vi "XboxTeleop.vi"(10 "Match Info":T1={"Autonomous Elapsed Seconds"=0.0, "TeleOp Elapsed Seconds"=0.0, "Disabled Elapsed Seconds"=0.0, "Visited Autonomous"=FALSE, "Visited TeleOp"=FALSE, "Visited Disabled"=FALSE, "Autonomous Settings"={"Autonomous Style"=enum."Independent", "VI Refnum"=refnum}}, 11 "Call Context":T2) -> ()   [LabVIEW 2015]
doc: "This VI is called for each TeleOp packet received from the DS where the robot is not disabled. It is often used to read from the joysticks and update I/O or to update setpoints for timed control loops. It should complete and return within 20 milliseconds or it may miss DS packets."
uses:
  <vilib>/Rock Robotics/WPI/DriverStation/WPI_DriverStationDerivedRobotMode.ctl
  <vilib>/Rock Robotics/WPI/DriverStation/WPI_DriverStationMatch Info.ctl
  <vilib>/Rock Robotics/WPI/Utilities/WPI_GetSetVariantRefNum.vi
  <vilib>/Rock Robotics/Network Tables/NT Write Boolean Array.vi
  <vilib>/Rock Robotics/Network Tables/NT Write Numeric Array.vi
  <vilib>/Rock Robotics/Network Tables/NT Write Boolean.vi
  <vilib>/Rock Robotics/Network Tables/NT Read Boolean.vi
  <vilib>/Rock Robotics/Network Tables/NT Read Number.vi
  <vilib>/Rock Robotics/WPI/RobotDrive/WPI_RobotDriveArcadeDrive_Standard(NoSaturation).vi
panel:
  in  "TurnPercent":dbl=0.9 format="%#_13g"
  out "TurnOutput":dbl(slide) scale=-1.0..1.0
  out "MotorInput":dbl(knob) scale=-1.0..1.0
  in  "DrivePercent":dbl=0.75 format="%#_13g"
  out "Sample Slider 0":dbl(slide) scale=0.0..5.0
  out "Sample Boolean 1":bool
  out "Sample Boolean 0":bool
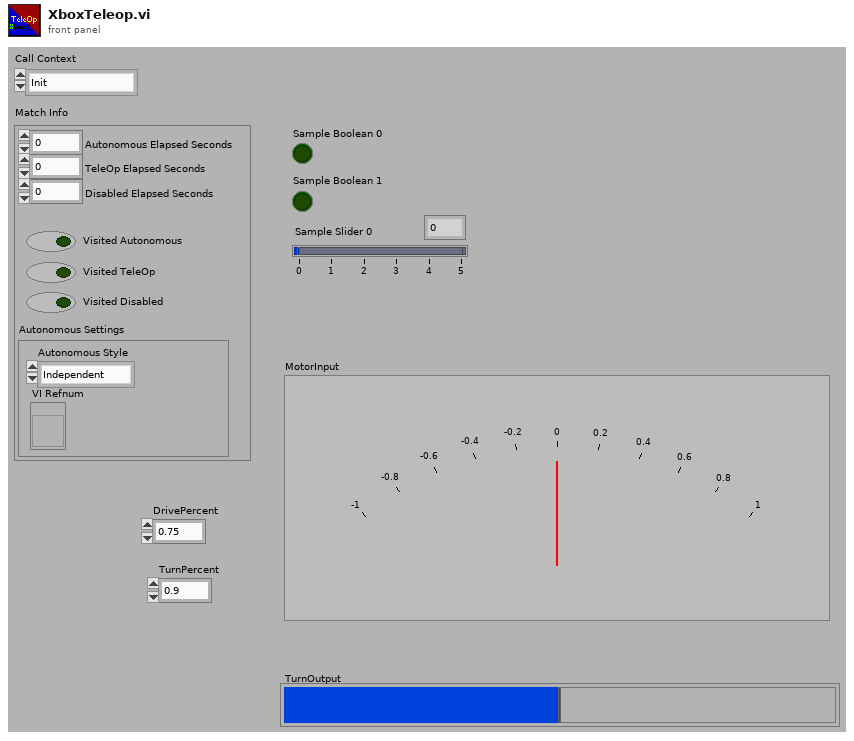
[diagram p1: front panel]
types:
  T1 = typedef "WPI_DriverStationMatch Info.ctl" = cluster{"Autonomous Elapsed Seconds":dbl, "TeleOp Elapsed Seconds":dbl, "Disabled Elapsed Seconds":dbl, "Visited Autonomous":bool, "Visited TeleOp":bool, "Visited Disabled":bool, "Autonomous Settings":cluster{"Autonomous Style":enum16{"Iterative", "Independent"}, "VI Refnum":refnum<vi>}}
  T2 = typedef "WPI_DriverStationDerivedRobotMode.ctl" = enum16{"Init", "Execute", "Stop"}
  T3 = typedef "WPI_RobotDriveDevRef.ctl" = cluster{"DevStatus":errorcluster, "Motors[]":T4[], "Square Inputs":bool, "Max Output":dbl}
  T4 = typedef "WPI_MotorControlDeviceRef.ctl" = cluster{"DeviceStatus":errorcluster, "Type":T5, "PWM":cluster{"PWM Channel":T6, "DeadBand":T7}, "CAN":cluster{"Device Number":u8, "Control Mode":T8, "Semaphore":T9, "Max Vout":dbl, "TalonSRX Control Mode":T10}, "Invert":bool}
  T5 = typedef "WPI_MotorControlType.ctl" = enum16{"PWM", "CAN", "CANTalonSRX"}
  T6 = typedef "FPGA_DIOPWMChannel.ctl" = enum8{"PWM 0", "PWM 1", "PWM 2", "PWM 3", "PWM 4", "PWM 5", "PWM 6", "PWM 7", "PWM 8", "PWM 9", "PWM MXP 0", "PWM MXP 1", "PWM MXP 2", "PWM MXP 3", "PWM MXP 4", "PWM MXP 5", "PWM MXP 6", "PWM MXP 7", "PWM MXP 8", "PWM MXP 9", "Invalid"}
  T7 = typedef "WPI_PWMDeadband.ctl" = cluster{"Name":string, "maxPositivePwm":i32, "minPositivePwm":i32, "centerPwm":i32, "maxNegativePwm":i32, "minNegativePwm":i32, "angularRange":u16}
  T8 = typedef "WPI_CANJaguar_ControlMode.ctl" = enum8{"Percent VBus", "Current", "Speed", "Position", "Voltage"}
  T9 = typedef "Semaphore RefNum" = refnum<k1>
  T10 = typedef "WPI_CANTalonSRX_APIControlMode.ctl" = enum8{"Percent VBus", "Speed", "Position", "Slave", "Unchanged / Invalid", "Voltage Compensation", "Current", "Motion Profile"}
  T11 = typedef "WPI_JoystickDevRef.ctl" = cluster{"Device":T12}
  T12 = typedef "WPI_JoystickDeviceEnum.ctl" = enum16{"USB 0", "USB 1", "USB 2", "USB 3", "USB 4", "USB 5"}
  T13 = cluster{"Buttons[0]":bool, "Buttons[1]":bool, "Buttons[2]":bool, "Buttons[3]":bool, "Buttons[4]":bool, "Buttons[5]":bool, "Buttons[6]":bool, "Buttons[7]":bool, "Buttons[8]":bool}
  T14 = cluster{"Axes[0]":dbl, "Axes[1]":dbl, "Axes[2]":dbl, "Axes[3]":dbl, "Axes[4]":dbl, "Axes[5]":dbl, "Axes[6]":dbl, "Axes[7]":dbl, "Axes[8]":dbl}
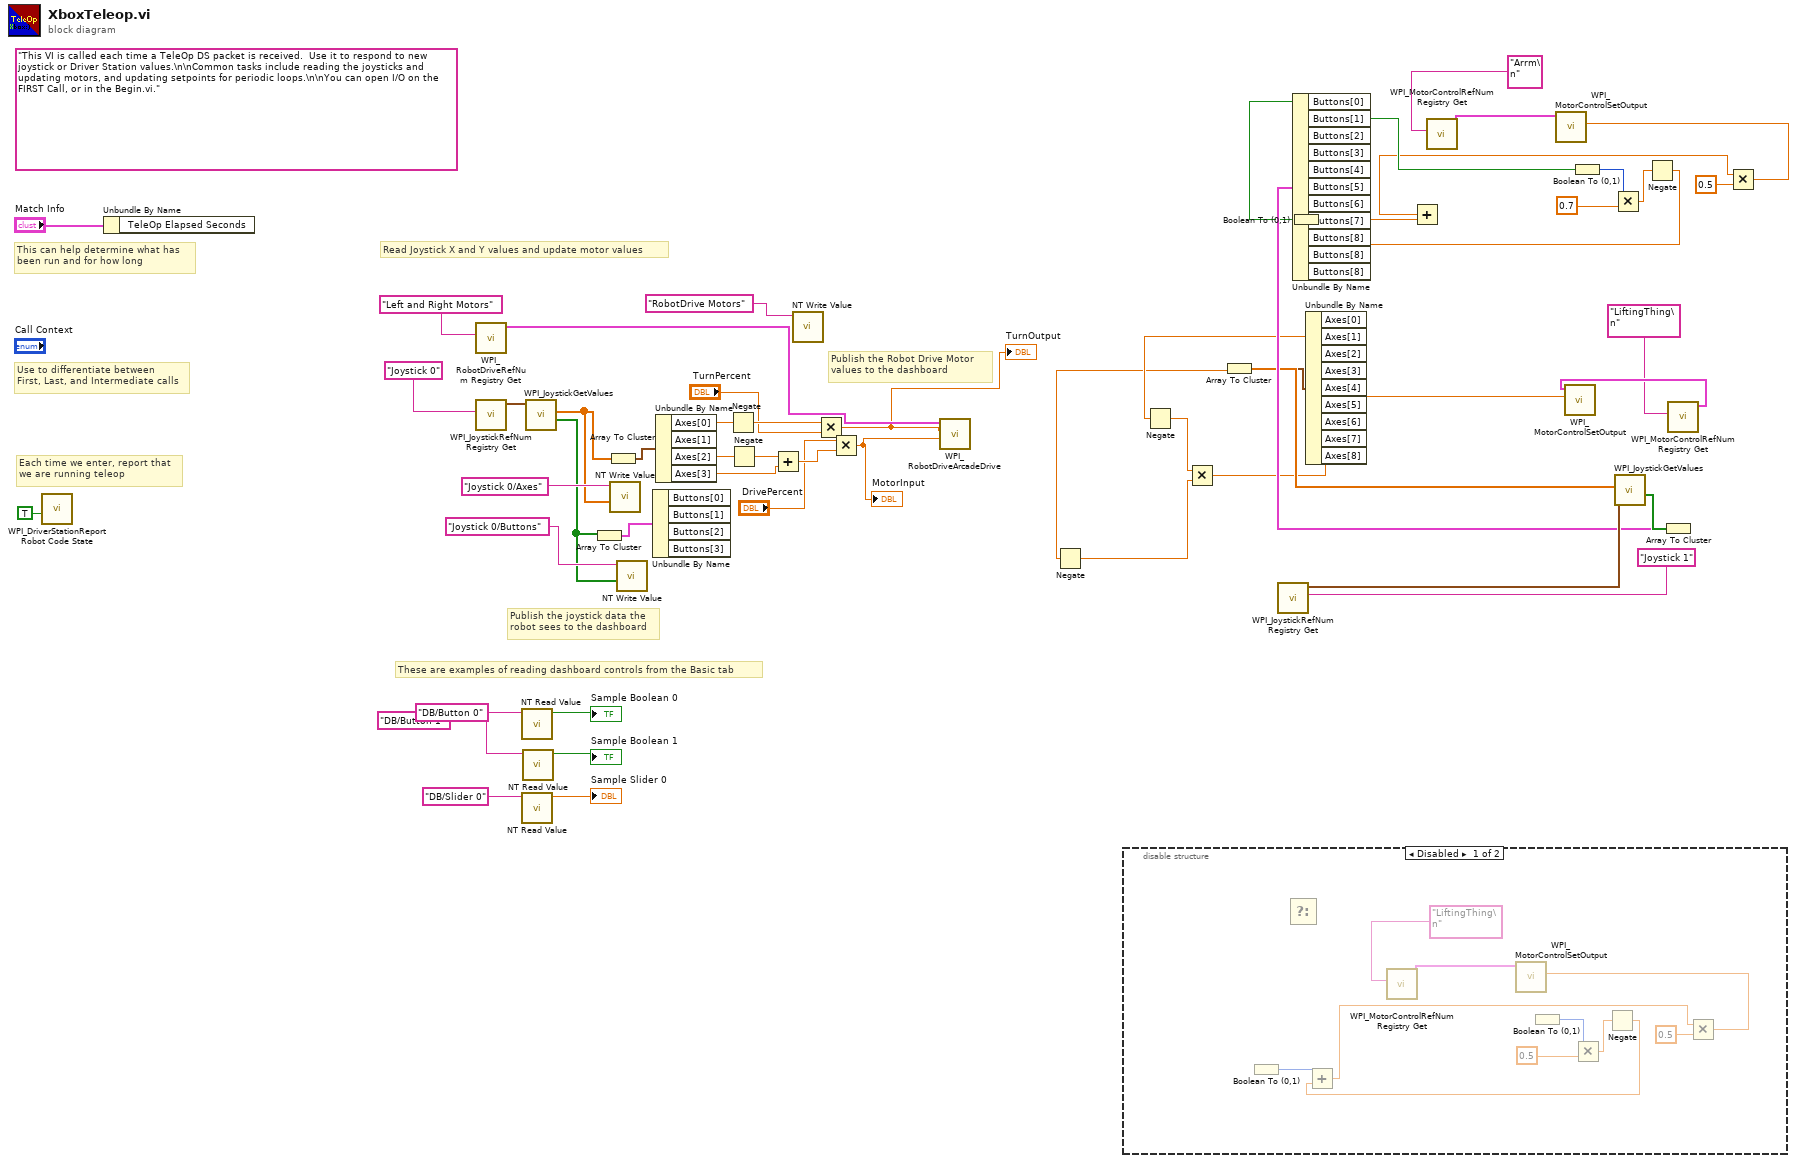
[diagram p0: block diagram]
diagram:
  (unwired) "This VI is called each time a TeleOp DS packet is received.  Use it to respond to new joystick or Driver Station values.\n\nCommon tasks include reading the joysticks and updating motors, and updating setpoints for periodic loops.\n\nYou can open I/O on the FIRST Call, or in the Begin.vi."
  # "These are examples of reading dashboard controls from the Basic tab"
  # "Publish the Robot Drive Motor\nvalues to the dashboard"
  # "Publish the joystick data the\nrobot sees to the dashboard"
  # "Each time we enter, report that\nwe are running teleop"
  # "Use to differentiate between\nFirst, Last, and Intermediate calls"
  # "This can help determine what has\nbeen run and for how long"
  # "Read Joystick X and Y values and update motor values"
  n1 = call <vilib>:"WPI_DriverStationReport Robot Code State.vi"("TeleOp"=TRUE ("Autonomous")) -> ()  [unwired: 10 in, 1 out]
  n2 = Unbundle By Name("Match Info") -> ()  [unwired: 1 out]
  n3 = call <vilib>:"WPI_RobotDriveRefNum Registry Get.vi"("refnum name"="Left and Right Motors") -> ("RobotDriveDevRef"=w38:T3)  [unwired: 1 in, 9 out]
  n4 = call <vilib>:"WPI_JoystickRefNum Registry Get.vi"("refnum name"="Joystick 0") -> ("JoystickDevRef"=w51:T11)  [unwired: 1 in, 9 out]
  n5 = call-poly <vilib>:"NT Read Value.vi"("Name"="DB/Button 0" ("refnum name")) -> ("Boolean"=→"Sample Boolean 0":bool)  [unwired: 9 in, 1 out]
  n6 = call-poly <vilib>:"NT Read Value.vi"("Name"="DB/Slider 0" ("refnum name")) -> ("Numeric"=→"Sample Slider 0":dbl)  [unwired: 9 in, 1 out]
  n7 = call-poly <vilib>:"NT Read Value.vi"("Name"="DB/Button 1" ("refnum name")) -> ("Boolean"=→"Sample Boolean 1":bool)  [unwired: 9 in, 1 out]
  n8 = call <vilib>:"WPI_JoystickGetValues.vi"("JoystickDevRef"=w51) -> ("Buttons"=w36:bool[], "Axes"=w39:dbl[])  [unwired: 6 in, 3 out]
  n9 = Array To Cluster(array=w36) -> (cluster=w35:T13)
  n10 = Array To Cluster(array=w39) -> (cluster=w40:T14)
  n11 = call-poly <vilib>:"NT Write Value.vi"("Numeric Array"=w39, "Name"="Joystick 0/Axes") -> ()  [unwired: 9 in, 1 out]
  n12 = call-poly <vilib>:"NT Write Value.vi"("Boolean Array"=w36, "Name"="Joystick 0/Buttons") -> ()  [unwired: 9 in, 1 out]
  n13 = Unbundle By Name(w35) -> ()  [unwired: 4 out]
  n14 = Unbundle By Name(w40) -> ("Axes[0]"=w37:dbl, "Axes[2]"=w34:dbl, "Axes[3]"=w32:dbl)  [unwired: 1 out]
  n15 = Negate(x=w37) -> (-x=w29:dbl)
  n16 = Negate(x=w34) -> (-x=w33:dbl)
  n17 = Add(x=w33, y=w32) -> (x+y=w31:dbl)
  n18 = call-poly <vilib>:"NT Write Value.vi"("Name"="RobotDrive Motors") -> ()  [unwired: 10 in, 1 out]
  n19 = Multiply(x=w29, y="TurnPercent") -> (x*y=w28:dbl)
  "TurnOutput" <- w28
  n20 = Multiply(x="DrivePercent", y=w31) -> (x*y=w30:dbl)
  "MotorInput" <- w30
  n21 = call-poly <vilib>:"WPI_RobotDriveArcadeDrive.vi"("Y axis value"=w30, "X axis value"=w28, "RobotDriveDevRef"=w38) -> ()  [unwired: 6 in, 3 out]
  n22 = disable-structure shown="Disabled" {
    frame Disabled {
      n23 = Boolean To (0,1)() -> (0, 1=w63:i16)  [unwired: 1 in]
      n24 = Select() -> ()  [unwired: 3 in, 1 out]
      n25 = call <vilib>:"WPI_MotorControlRefNum Registry Get.vi"("refnum name"="LiftingThing\n") -> ("MotorControlDevRef"=w59:T4)  [unwired: 9 in, 1 out]
      n26 = Boolean To (0,1)() -> (Boolean=w65:bool, 0, 1=w62:i16)
      n27 = Multiply(x=w62, y=0.5) -> (x*y=w61:dbl)
      n28 = Negate(x=w61) -> (-x=w64:dbl)
      n29 = Add(x=w63, y=w64) -> (x+y=w57:dbl)
      n30 = Multiply(x=w57, y=0.5) -> (x*y=w56:dbl)
      n31 = call <vilib>:"WPI_MotorControlSetOutput.vi"("Output"=w56, "MotorControlDevRef"=w59) -> ()  [unwired: 7 in, 3 out]
    }
    frame Enabled {
    }
  }
  n32 = call <vilib>:"WPI_JoystickRefNum Registry Get.vi"("refnum name"="Joystick 1") -> ("JoystickDevRef"=w24:T11)  [unwired: 1 in, 9 out]
  n33 = call <vilib>:"WPI_MotorControlRefNum Registry Get.vi"("refnum name"="Arrm\n") -> ("MotorControlDevRef"=w14:T4)  [unwired: 9 in, 1 out]
  n34 = call <vilib>:"WPI_JoystickGetValues.vi"("JoystickDevRef"=w24) -> ("Buttons"=w23:bool[], "Axes"=w9:dbl[])  [unwired: 6 in, 3 out]
  n35 = Array To Cluster(array=w9) -> (cluster=w8:T14)
  n36 = Unbundle By Name(w8) -> ("Axes[1]"=w4:dbl, "Axes[3]"=w2:dbl)  [unwired: 7 out]
  n37 = Negate(x=w2) -> (-x=w1:dbl)
  n38 = Negate(x=w4) -> (-x=w3:dbl)
  n39 = Multiply(x=w3, y=w1) -> (x*y=w5:dbl)
  n40 = Array To Cluster(array=w23) -> (cluster=w22:T13)
  n41 = Unbundle By Name(w22) -> ("Buttons[0]"=w21:bool, "Buttons[1]"=w20:bool)  [unwired: 9 out]
  n42 = Boolean To (0,1)(Boolean=w21) -> (0, 1=w18:i16)
  n43 = Boolean To (0,1)(Boolean=w20) -> (0, 1=w17:i16)
  n44 = Multiply(x=w17, y=0.7) -> (x*y=w16:dbl)
  n45 = Negate(x=w16) -> (-x=w19:dbl)
  n46 = Add(x=w18, y=w19) -> (x+y=w12:dbl)
  n47 = call <vilib>:"WPI_MotorControlRefNum Registry Get.vi"("refnum name"="LiftingThing\n") -> ("MotorControlDevRef"=w7:T4)  [unwired: 9 in, 1 out]
  n48 = call <vilib>:"WPI_MotorControlSetOutput.vi"("Output"=w5, "MotorControlDevRef"=w7) -> ()  [unwired: 7 in, 3 out]
  n49 = Multiply(x=w12, y=0.5) -> (x*y=w11:dbl)
  n50 = call <vilib>:"WPI_MotorControlSetOutput.vi"("Output"=w11, "MotorControlDevRef"=w14) -> ()  [unwired: 7 in, 3 out]
